vi "CONEX-LDS Get Laser Power Enable v2.vi"(11 "Connection Cluster in":T1) -> (1 "Laser Enabled (0 = F, 1 = T)":dbl, 3 "Connection Cluster out":T1)   [LabVIEW 2010]
doc: "LB? - Get Laser Power Enabled\n\nOutput: Laser Enabled state value"
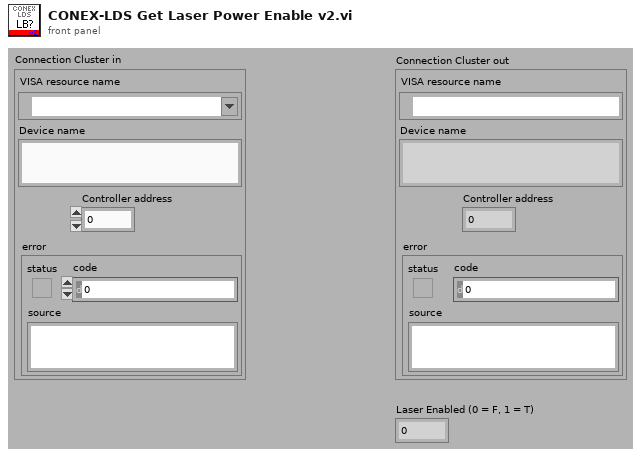
[diagram p1: front panel]
types:
  T1 = cluster{"VISA resource name":refnum<visa-resource-name>, "Device name":string, "Controller address":i32, "error":errorcluster}
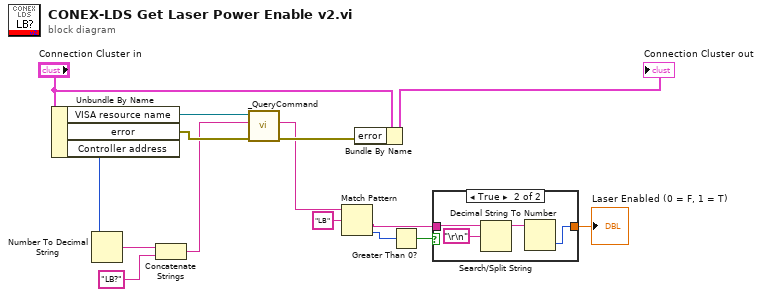
[diagram p0: block diagram]
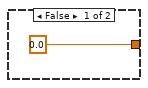
[diagram p2: hidden frame]
diagram:
  n1 = Unbundle By Name("Connection Cluster in") -> ("VISA resource name"=w8:refnum<visa-resource-name>, "error"=w7:errorcluster, "Controller address"=w3:i32)
  n2 = Number To Decimal String(number=w3) -> (decimal integer string=w15:string)  [unwired: 1 out]
  n3 = Concatenate Strings(w15, "LB?" ("strCommand")) -> (w2:string)
  n4 = call <userlib>:"_QueryCommand.vi"("error in"=w7, "Command"=w2, "Instrument Channel in"=w8) -> ("error out"=w5:errorcluster, "Response"=w1:string)  [unwired: 6 in, 1 out]
  n5 = Match Pattern(string=w1, regular expression="LB" ("expression régulière")) -> (after substring=w12:string, offset past match=w11:i32)  [unwired: 3 out]
  n6 = Bundle By Name(cluster="Connection Cluster in", "error"=w5) -> (→"Connection Cluster out":T1)
  n7 = Greater Than 0?(x=w11) -> (x > 0?=w10:bool)
  n8 = case shown="True" w10 {
    tunnel: w12 -> [_ w19]
    tunnel: [0.0 w17] -> w9
    frame False {
    }
    frame True {
      n9 = Search/Split String(string=w19, search string/char (-)="\r\n") -> (substring before match=w18:string)  [unwired: 3 out]
      n10 = Decimal String To Number(string=w18) -> (number=w17:i32)  [unwired: 2 in, 1 out]
    }
  }
  "Laser Enabled (0 = F, 1 = T)" <- w9
